vi "Analyze Data.vi"(8 "error in":errorcluster, 11 "CRDS in":refnum<class "CRDS.lvclass">) -> (0 "error out":errorcluster, 3 "CRDS out":refnum<class "CRDS.lvclass">)   [LabVIEW 2017, in "CRDS Lib.lvlib" / "CRDS.lvclass"]
doc: "Analyze Data takes the stored ringdown data (1000 shots per cell) and:\n1) Calculates the ringdown decay constant tau\n2) Averages tau0 data as necessary\n3) Corrects the tau data for Rayleigh scattering\n4) Stores a 1-D array of taus returned on a 1 kHz basis (8k taus) if a jump drive (U:) is connected\n5) Flattens the data into a string and stuffs the string into the <b>data</b> shared variable for display on the UI.\n\nThis VI will not be called if the data is not \"good\" (that is, if an error was thrown in the <B>Get Data</B> routine. If an error is thrown while the data is being retrieved, then the data will not be sent to the UI."
uses:
  CRDS.lvclass
  Z:/sw_repo/For Builds/Reusable/Instrument/Instrument.lvclass
  Instrument/Instrument.lvclass/Instrument.ctl
  CRDS.lvclass/CRDS.ctl
  Data/Main/CRDS Data.lvclass
  Z:/sw_repo/For Builds/Reusable/Data/Data.lvclass
  Cell/CRDS Cell.lvclass/CRDS Cell.ctl
  Data/Cell/CRDS Cell Data.lvclass/CRDS Cell Data.ctl
  Cell/Read Laser Data.vi
  Data/Cell/Write Laser Data.vi
  Instrument/Write Data.vi
  Read Saving RDs.vi
  Read Cells.vi
  Write Cells.vi
  Data/Data.lvclass
  Cell/CRDS Cell.lvclass
  Data/Cell/CRDS Cell Data.lvclass
  Instrument/Instrument.lvclass
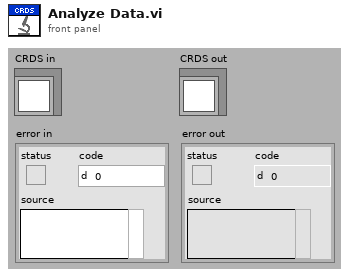
[diagram p1: front panel]
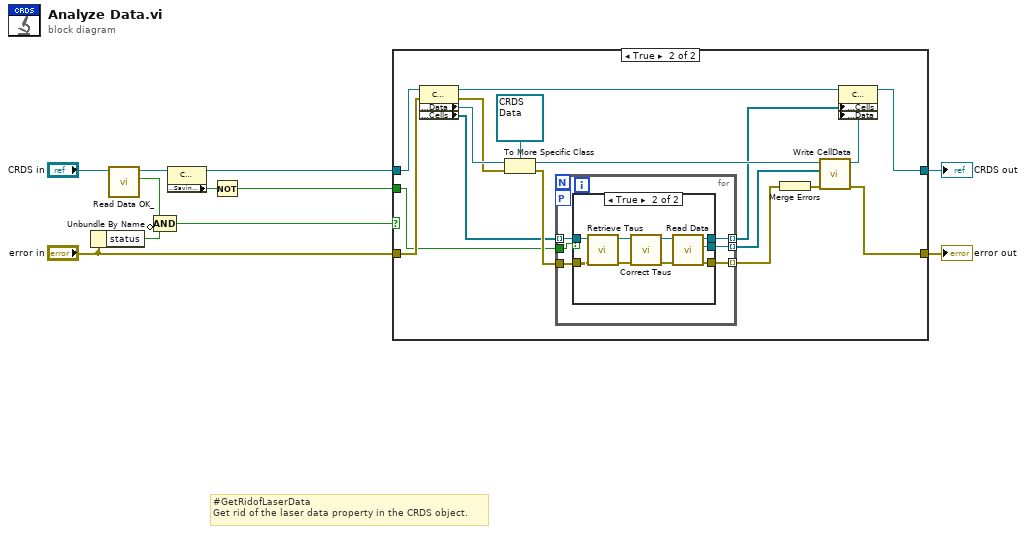
[diagram p0: block diagram]
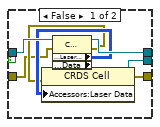
[diagram p3: hidden frame]
diagram:
  # "#GetRidofLaserData\nGet rid of the laser data property in the CRDS object."
  n1 = Unbundle By Name("error in") -> ("status"=w3:bool)
  n2 = call "Read Data OK_.vi"("Instrument in"="CRDS in") -> ("Data OK?"=w4:bool, "Instrument out"=w7:refnum<class "CRDS.lvclass">)  [unwired: 8 in, 1 out]
  n3 = Compound Arithmetic op=AND(w4, invert w3) -> (w2:bool)
  n4 = property class="CRDS"(reference=w7) -> (reference out=w6:refnum<class "CRDS.lvclass">, "Data Access:Saving RDs"=w5:bool)  [unwired: 1 in, 1 out]
  n5 = Not(x=w5) -> (.not. x?=w1:bool)
  n6 = case shown="True" w2 {
    tunnel: w6 -> [w13 w29]
    tunnel: "error in" -> [w12 w16]
    tunnel: [w13 w27] -> w10
    tunnel: [w12 w30] -> w9
    tunnel: w1 -> [_ w14]
    frame False {
    }
    frame True {
      n7 = property class="CRDS"(reference=w29, error in=w16) -> (reference out=w18:refnum<class "CRDS.lvclass">, error out=w15:errorcluster, "Accessors:Data"=w21:refnum<class "Data.lvclass">, "Data Access:Cells"=w17:refnum<class "CRDS Cell.lvclass">[])
      n8 = To More Specific Class(target class=refnum<class "CRDS Data.lvclass"> refnum ("reference out"), reference=w21, error in=w15) -> (specific class reference=w22:refnum<class "CRDS Data.lvclass">, error out=w24:errorcluster)
      n9 = for "Initial extinction calculation" {
        tunnel: w17 -> [w36] mode=indexing
        tunnel: w24 -> [w32]
        tunnel: [w35] -> w20 mode=indexing
        tunnel: [w34] -> w26 mode=indexing
        tunnel: [w33] -> w25 mode=indexing
        workers-P: _ -> [_]
        tunnel: w14 -> [w31]
        n10 = case shown="True" w31 {
          tunnel: w36 -> [w44 w51]
          tunnel: [w42 w48] -> w35
          tunnel: [w43 w47] -> w34
          tunnel: [w40 w46] -> w33
          tunnel: w32 -> [w37 w45]
          frame False {
            n11 = property class="CRDS Cell"(reference=w44, error in=w37) -> (reference out=w42:refnum<class "CRDS Cell.lvclass">, error out=w38:errorcluster, "Accessors:Laser Data"=w39:i16[][], "Accessors:Data"=w41:refnum<class "CRDS Cell Data.lvclass">)
            n12 = property class="CRDS Cell"(reference=w41, error in=w38, "Accessors:Laser Data"=w39) -> (reference out=w40:refnum<class "CRDS Cell Data.lvclass">, error out=w43:errorcluster)
          }
          frame True {
            n13 = call "Retrieve Taus.vi"("error in"=w45, "CRDS Cell in"=w51) -> ("error out"=w52:errorcluster, "CRDS Cell out"=w53:refnum<class "CRDS Cell.lvclass">)  [unwired: 7 in, 1 out]
            n14 = call "Correct Taus.vi"("error in"=w52, "CRDS Cell in"=w53) -> ("error out"=w49:errorcluster, "CRDS Cell out"=w50:refnum<class "CRDS Cell.lvclass">)  [unwired: 8 in]
            n15 = call "Read Data.vi"("error in"=w49, "CRDS Cell in"=w50) -> ("error out"=w47:errorcluster, "CRDS Cell"=w46:refnum<class "CRDS Cell Data.lvclass">, "CRDS Cell out"=w48:refnum<class "CRDS Cell.lvclass">)  [unwired: 7 in]
          }
        }
      }
      n16 = Merge Errors(w26) -> (w23:errorcluster)
      n17 = call "Write CellData.vi"("error in"=w23, "CellData"=w25, "CRDS Data in"=w22) -> ("error out"=w30:errorcluster, "CRDS Data out"=w19:refnum<class "CRDS Data.lvclass">)  [unwired: 7 in]
      n18 = property class="CRDS"(reference=w18, "Data Access:Cells"=w20, "Accessors:Data"=w19) -> (reference out=w27:refnum<class "CRDS.lvclass">)  [unwired: 1 in, 1 out]
    }
  }
  "error out" <- w9
  "CRDS out" <- w10
